vi "Advantech.vi"(8 "error in (no error)":errorcluster, 11 "TC Coefficients":T1) -> (0 "error out":errorcluster, 3 "Advantech":T2, 5 "Avantech DAQ":string[][](array[string]), 7 "Parametric DBL Data":dbl[](array[numeric]))   [LabVIEW 2014]
uses:
  Type Definitions/AdvantechDAQ.ctl
  Type Definitions/TC Coefficients.ctl
  Type Definitions/TC Coefficients Selector.ctl
panel:
  out "Raw Data":dbl[](array[numeric])
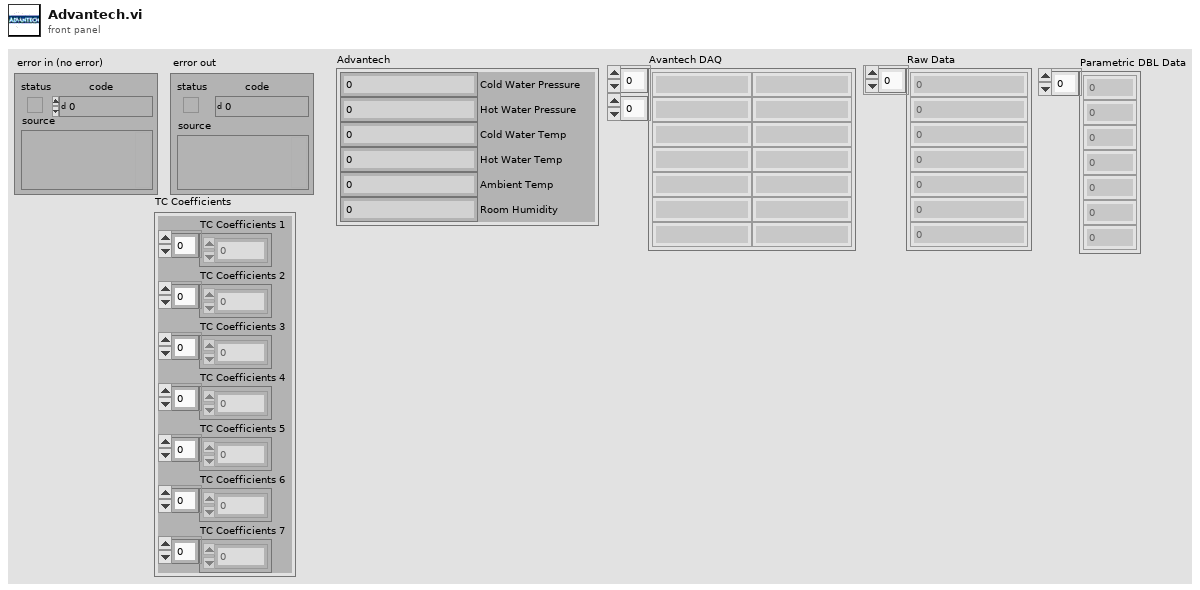
[diagram p1: front panel]
types:
  T1 = typedef "TC Coefficients.ctl" = cluster{"TC Coefficients 1":dbl[], "TC Coefficients 2":dbl[], "TC Coefficients 3":dbl[], "TC Coefficients 4":dbl[], "TC Coefficients 5":dbl[], "TC Coefficients 6":dbl[], "TC Coefficients 7":dbl[]}
  T2 = typedef "AdvantechDAQ.ctl" = cluster{"Cold Water Pressure":dbl, "Hot Water Pressure":dbl, "Cold Water Temp":dbl, "Hot Water Temp":dbl, "Ambient Temp":dbl, "Room Humidity":dbl}
  T3 = typedef "TC Coefficients Selector.ctl" = enum16{"TC1", "TC2", "TC3", "TC4", "TC5", "TC6", "TC7"}
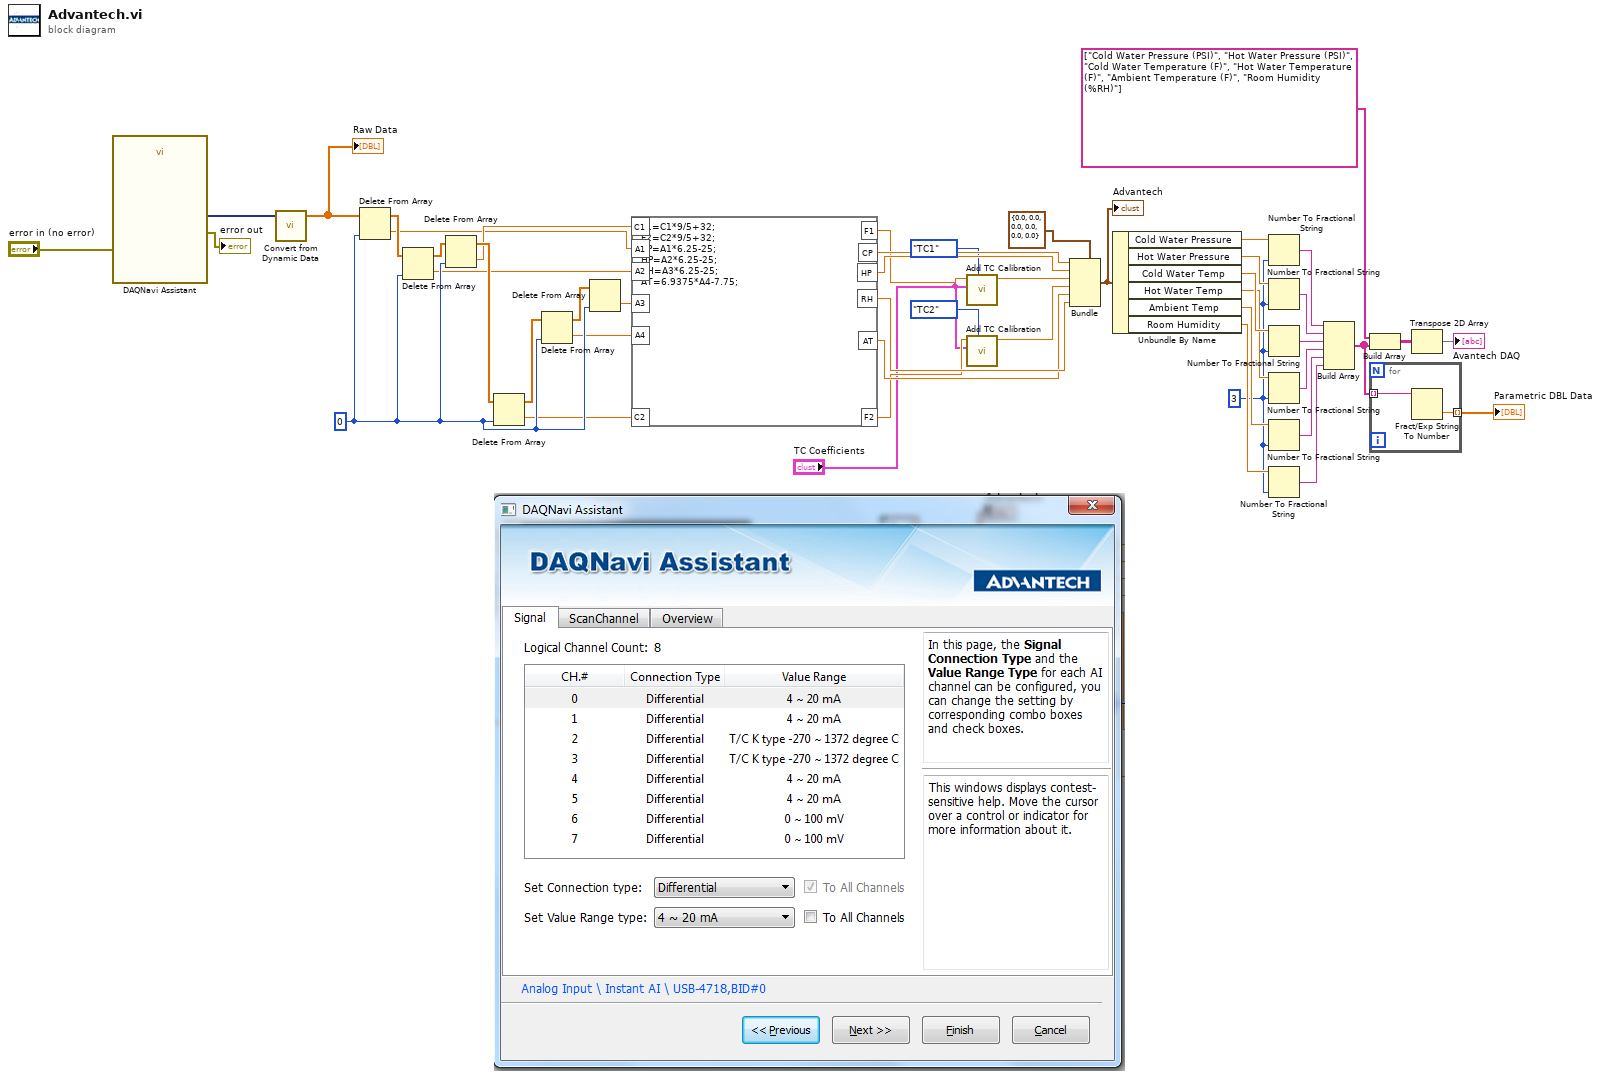
[diagram p0: block diagram]
diagram:
  w8 = i16 3 ("precision (6)")
  w38 = 0 ("index")
  n1 = call "DAQNavi Assistant"("error in(no error)"="error in (no error)") -> ("error out"=→"error out":errorcluster, "data out(DDT)"=w45:dynamicdata)  [unwired: 17 in]
  n2 = call "Convert from Dynamic Data"("Dynamic Data Type"=w45) -> ("Array"=w44:dbl[])  [unwired: 3 in]
  "Raw Data" <- w44
  n3 = Delete From Array(array=w44, index=w38) -> (deleted portion=w35:dbl, array with subset deleted=w43:dbl[])  [unwired: 1 in]
  n4 = Delete From Array(array=w43, index=w38) -> (deleted portion=w31:dbl, array with subset deleted=w42:dbl[])  [unwired: 1 in]
  n5 = Delete From Array(array=w42, index=w38) -> (deleted portion=w37:dbl, array with subset deleted=w41:dbl[])  [unwired: 1 in]
  n6 = Delete From Array(array=w41, index=w38) -> (deleted portion=w36:dbl, array with subset deleted=w40:dbl[])  [unwired: 1 in]
  n7 = Delete From Array(array=w40, index=w38) -> (deleted portion=w29:dbl, array with subset deleted=w39:dbl[])  [unwired: 1 in]
  n8 = Delete From Array(array=w39, index=w38) -> (deleted portion=w34:dbl)  [unwired: 1 in, 1 out]
  n9 = formula code="F1=C1*9/5+32;\nF2=C2*9/5+32;\nCP=A1*6.25-25;\nHP=A2*6.25-25;\nRH=A3*6.25-25;\nAT=6.9375*A4-7.75;"("C1"=w37, "C2"=w36, "A1"=w35, "A2"=w31, "A3"=w34, "A4"=w29) -> ("F1"=w7:dbl, "F2"=w5:dbl, "CP"=w32:dbl, "HP"=w30:dbl, "RH"=w33:dbl, "AT"=w28:dbl)
  n10 = call "Add TC Calibration.vi"("Enum"=TC_Coefficients_Selector."TC1", "TC Coefficients"="TC Coefficients", "Non Cal Temp"=w7) -> ("Calibrated Temp"=w6:dbl)  [unwired: 8 in]
  n11 = call "Add TC Calibration.vi"("Enum"=TC_Coefficients_Selector."TC2", "TC Coefficients"="TC Coefficients", "Non Cal Temp"=w5) -> ("Calibrated Temp"=w4:dbl)  [unwired: 8 in]
  n12 = Bundle(cluster=T2 {"Cold Water Pressure"=0.0, "Hot Water Pressure"=0.0, "Cold Water Temp"=0.0, "Hot Water Temp"=0.0, "Ambient Temp"=0.0, "Room Humidity"=0.0} ("Advantech 2"), "Cold Water Pressure"=w32, "Hot Water Pressure"=w30, "Cold Water Temp"=w6, "Hot Water Temp"=w4, "Ambient Temp"=w28, "Room Humidity"=w33) -> (w27:T2)
  "Advantech" <- w27
  n13 = Unbundle By Name(w27) -> ("Cold Water Pressure"=w25:dbl, "Hot Water Pressure"=w24:dbl, "Cold Water Temp"=w23:dbl, "Hot Water Temp"=w22:dbl, "Ambient Temp"=w21:dbl, "Room Humidity"=w20:dbl)
  n14 = Number To Fractional String(number=w25, precision (6)=w8) -> (F-format string=w19:string)  [unwired: 2 in]
  n15 = Number To Fractional String(number=w24, precision (6)=w8) -> (F-format string=w18:string)  [unwired: 2 in]
  n16 = Number To Fractional String(number=w23, precision (6)=w8) -> (F-format string=w17:string)  [unwired: 2 in]
  n17 = Number To Fractional String(number=w22, precision (6)=w8) -> (F-format string=w16:string)  [unwired: 2 in]
  n18 = Number To Fractional String(number=w21, precision (6)=w8) -> (F-format string=w15:string)  [unwired: 2 in]
  n19 = Number To Fractional String(number=w20, precision (6)=w8) -> (F-format string=w14:string)  [unwired: 2 in]
  n20 = Build Array(w19, w18, w17, w16, w15, w14) -> (w10:string[])
  n21 = Build Array(string[] ["Cold Water Pressure (PSI)", "Hot Water Pressure (PSI)", "Cold Water Temperature (F)", "Hot Water Temperature (F)", "Ambient Temperature (F)", "Room Humidity (%RH)"], w10) -> (w12:string[][])
  n22 = for {
    tunnel: w10 -> [w49] mode=indexing
    tunnel: [w48] -> w9 mode=indexing
    n23 = Fract/Exp String To Number(string=w49) -> (number=w48:dbl)  [unwired: 3 in, 1 out]
  }
  "Parametric DBL Data" <- w9
  n24 = Transpose 2D Array(2D array=w12) -> (transposed array=→"Avantech DAQ":string[][])
